vi "ComputeRaster.vi"(6 "TestZT":cluster{"Z mm":dbl, "Horizontal T deg":dbl}, 7 "Polarization, V0 H1":T1, 9 "Position Array in":T2(array[cluster]), 10 "Window dimension":i32, 11 "Nyquist, mm":i32) -> (0 "Total points":dbl, 1 "XY Graph for evaluation":cluster{dbl[], dbl[]}[](array[cluster]), 2 "Position Array out":T3(array[cluster]), 3 "Window adjusted, cm":dbl)   [LabVIEW 2019]
doc: "The raster is computed based on the center of the four corner antenna postions.\nThe raster can be rotated in X and Y to align with the motion axes, or with the four corners (sides) of the antenna array."
uses:
  Classes/Sequence/SequenceSubvis/PolarizationSelect.ctl
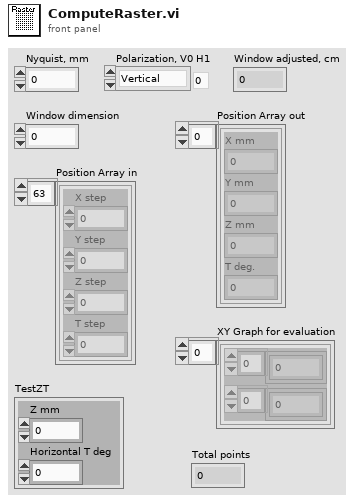
[diagram p1: front panel]
types:
  T1 = typedef "PolarizationSelect.ctl" = enum16{"Vertical", "Horizontal"}
  T2 = cluster{"X step":dbl, "Y step":dbl, "Z step":dbl, "T step":dbl}[]
  T3 = cluster{"X mm":dbl, "Y mm":dbl, "Z mm":dbl, "T deg.":dbl}[]
  T4 = cluster{"X step":dbl, "Y step":dbl, "Z step":dbl, "T step":dbl}
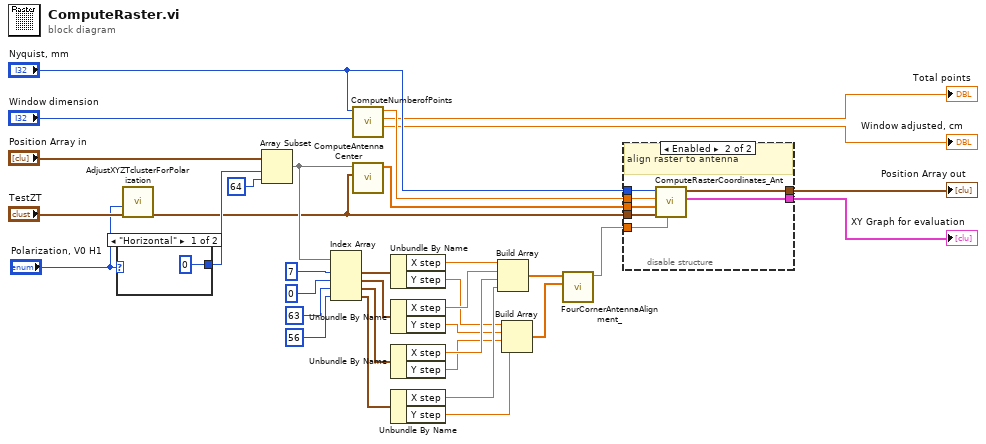
[diagram p0: block diagram]
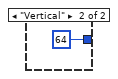
[diagram p2: hidden frame]
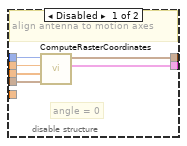
[diagram p3: hidden frame]
diagram:
  n1 = case shown="\"Horizontal\"" "Polarization, V0 H1" {
    tunnel: [0 ("index") 64 ("index")] -> w6
    frame "Horizontal" {
    }
    frame "Vertical" {
    }
  }
  n2 = call "AdjustXYZTclusterForPolarization.vi"("TestZT"="TestZT", "Polarization"="Polarization, V0 H1") -> ("TestZT out"=w3:cluster{"Z mm":dbl, "Horizontal T deg":dbl})  [unwired: 8 in, 1 out]
  n3 = Array Subset(array="Position Array in", index=w6, length=64 ("index")) -> (w5:T2)
  n4 = Index Array(array=w5, index #1=7 ("index"), index #2=0 ("index"), index #3=63 ("index"), index #4=56 ("index")) -> (element #1=w22:T4, element #2=w21:T4, element #3=w20:T4, element #4=w19:T4)
  n5 = call "ComputeNumberofPoints.vi"("Window, cm"="Window dimension", "Nyquist, mm"="Nyquist, mm") -> ("Window adjusted, cm"=→"Window adjusted, cm":dbl, "Total points"=→"Total points":dbl, "Points per side"=w32:dbl)  [unwired: 7 in]
  n6 = call "ComputeAntennaCenter.vi"("TestZT"=w3, "Motion64.ini Position Array"=w5) -> ("Solution Vector, y and x"=w30:dbl[])  [unwired: 8 in, 1 out]
  n7 = Unbundle By Name(w22) -> ("X step"=w18:dbl, "Y step"=w13:dbl)
  n8 = Unbundle By Name(w21) -> ("X step"=w17:dbl, "Y step"=w12:dbl)
  n9 = Unbundle By Name(w20) -> ("X step"=w16:dbl, "Y step"=w11:dbl)
  n10 = Unbundle By Name(w19) -> ("X step"=w14:dbl, "Y step"=w10:dbl)
  n11 = Build Array(w18, w17, w16, w14) -> (w15:dbl[])
  n12 = Build Array(w13, w12, w11, w10) -> (w9:dbl[])
  n13 = call "FourCornerAntennaAlignment_.vi"("Y corners, 7, 0, 63, 56"=w9, "X corners, 7, 0, 63, 56"=w15) -> ("x direction angle"=w8:dbl)  [unwired: 7 in, 2 out]
  n14 = disable-structure shown="Enabled" {
    disable-tunnel: w3 -> [w42 w49]
    disable-tunnel: [w41 w45] -> w34
    disable-tunnel: [w40 w44] -> w33
    disable-tunnel: w32 -> [w39 w47]
    disable-tunnel: "Nyquist, mm" -> [w38 w46]
    disable-tunnel: w30 -> [w37 w48]
    disable-tunnel: w8 -> [_ w43]
    frame Disabled {
      # "angle = 0"
      # "align antenna to motion axes"
      n15 = call "ComputeRasterCoordinates.vi"("TestZT"=w42, "Center Vector, y and x"=w37, "Points per side"=w39, "Nyquist, mm"=w38) -> ("XY Graph for evaluation"=w40:cluster{dbl[], dbl[]}[], "Raster Position Array"=w41:T3)  [unwired: 6 in]
    }
    frame Enabled {
      # "align raster to antenna"
      n16 = call "ComputeRasterCoordinates_Ant.vi"("antenna angle"=w43, "TestZT"=w49, "Center Vector, y and x"=w48, "Points per side"=w47, "Nyquist, mm"=w46) -> ("XY Graph for evaluation"=w44:cluster{dbl[], dbl[]}[], "Position Array"=w45:T3)  [unwired: 5 in]
    }
  }
  "Position Array out" <- w34
  "XY Graph for evaluation" <- w33
